vi "X Value.vi"() -> ()   [LabVIEW 2015]
panel:
  in  "X":dbl
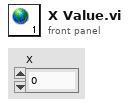
[diagram p1: front panel]
diagram:
